vi "WFS Calc Wavefront.vi"(8 "error in (no error)":errorcluster {"code" format="%.0x"}, 9 "Limit to Pupil (No)":i32(ring) items=["Yes"=1, "No"=0], 10 "Wavefront Type (Measured)":i32(ring) items=["Measured", "Reconstructed", "Difference"], 11 "instrument handle":refnum<visa-resource-name>) -> (0 "error out":errorcluster {"code" format="%.0x"}, 2 "Array Wavefront":sgl[](array[numeric]) format="%.2p", 3 "instrument handle out":refnum<visa-resource-name>)   [LabVIEW 2020]
doc: "This VI calculates the wavefront based on the spot deviations."
uses:
  WFS_32.dll
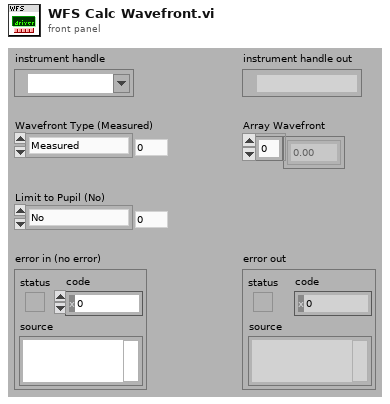
[diagram p1: front panel]
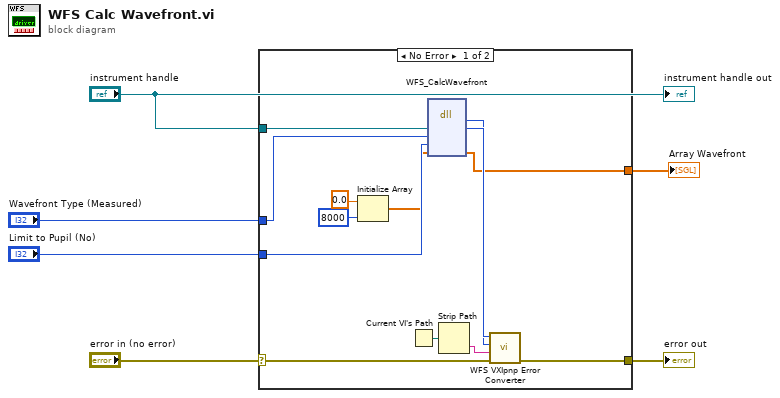
[diagram p0: block diagram]
diagram:
  n1 = case shown="No Error" "error in (no error)" {
    selector: "error in (no error)" -> [w14 w20]
    tunnel: [w13 w20] -> w6
    tunnel: "instrument handle" -> [w18 _]
    tunnel: "Wavefront Type (Measured)" -> [w12 _]
    tunnel: "Limit to Pupil (No)" -> [w11 _]
    tunnel: [w7 _] -> w1
    frame No Error {
      n2 = Initialize Array(sgl 0.0 ("element"), 8000 ("dimension size")) -> (w10:sgl[])
      n3 = Current VI's Path() -> (path=w19:path)
      n4 = dll-call lib="WFS_*.*" fn="WFS_CalcWavefront"("Instrument Handle"=w18, "Wavefront Type"=w12, "Limit to Pupil"=w11, "Array Wavefront"=w10) -> (w16:i32, "Instrument Handle"=w17:u32, "Array Wavefront"=w7:sgl[])  [unwired: 5 in, 2 out]
      n5 = Strip Path(path=w19) -> (name=w15:string)  [unwired: 1 out]
      n6 = call "WFS VXIpnp Error Converter.vi"("error in (no error)"=w14, "Name Of VI (\"\")"=w15, "CVI Error Code (0)"=w16, "instrument handle"=w17) -> ("error out"=w13:errorcluster)  [unwired: 6 in, 1 out]
    }
    frame Error {
    }
  }
  "error out" <- w6
  "Array Wavefront" <- w1
  "instrument handle out" <- "instrument handle"
